vi "FPGA_TANK_PRESS.vi"() -> ()   [LabVIEW 2018]
uses:
  <vilib>/LabVIEW Targets/FPGA/cRIO/shared/nicrio_ModuleControls/nicrio_cRIO-9205_VoltageRange.ctl
  <vilib>/LabVIEW Targets/FPGA/cRIO/shared/nicrio_ModuleControls/nicrio_cRIO-9205_TerminalMode.ctl
  <vilib>/rvi/Emulation/niFpgaGetClockAttributes.vi
  <vilib>/rvi/Emulation/niFpgaSctlEmulationGetInTimedLoop.vi
  <vilib>/rvi/Emulation/niFpgaEmulationReportErrorSimple.vi
  <vilib>/rvi/eio/common/nirviEmuTemplateMethod_errors.vi
  <vilib>/rvi/interface/RandomDataEmulation/niFpgaRandomDataHandleErrors.vi
  <vilib>/rvi/Emulation/niFpgaCriticalErrorInLSC.vi
  <vilib>/eio/EIOMethodNode/EIOMethodNode.xnode
  <vilib>/eio/EIONode/EIONode.xnode
  <vilib>/rvi/DataTransferAndStorage/Container/XNode/niFpgaContainer.xnode
  <vilib>/rvi/interface/RandomDataEmulation/nirviRandomDataFpgaReadWriteTemplate.vi
panel:
  out "Mod1/AI3":fxp<+/-,26,5>
  out "Mod1/AI2":fxp<+/-,26,5>
  out "Mod1/AI1":fxp<+/-,26,5>
  in  "Loop Rate (uS) 2":u32=4000
  out "Mod1/DI0":bool
  in  "Mod1/DO0 2":bool
  out "Mod1/AI0":fxp<+/-,26,5>
  in  "stop":bool
  out "FPGA Error Out 2":errorcluster
  in  "Mod2/DO0":bool
  in  "Mod2/DO3":bool
  in  "Mod2/DO2":bool
  in  "Mod2/DO1":bool
  in  "Mod2/DO4":bool
  in  "Mod2/DO7":bool
  in  "Mod2/DO6":bool
  in  "Mod2/DO5":bool
  in  "Stop":bool
  in  "Loop Rate (uS)":u32
  out "FPGA Error Out":errorcluster
  out "Data FIFO Full":bool
  in  "Update AI Settings":bool
  in  "AI Channel Settings":T3(array[cluster])=[{"Voltage Range"=enum."+/- 10V", "Terminal Mode"=enum."RSE"}, {"Voltage Range"=enum."+/- 10V", "Terminal Mode"=enum."RSE"}, {"Voltage Range"=enum."+/- 10V", "Terminal Mode"=enum."RSE"}, {"Voltage Range"=enum."+/- 10V", "Terminal Mode"=enum."RSE"}]
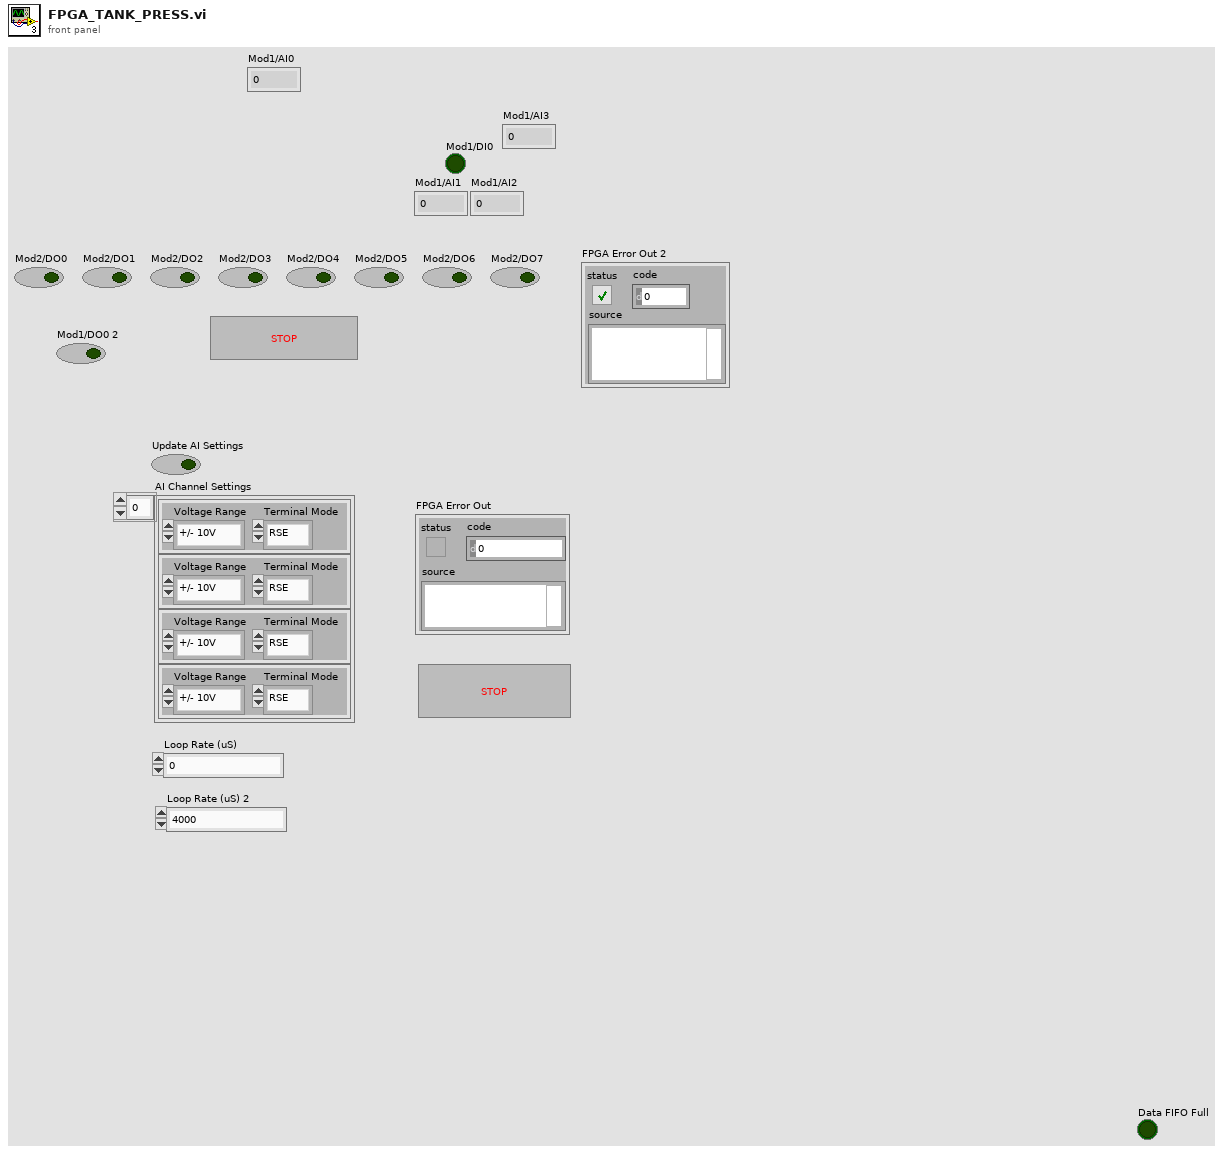
[diagram p1: front panel]
types:
  T1 = typedef "nicrio_cRIO-9205_VoltageRange.ctl" = enum8{"+/- 10V", "+/- 5V", "+/- 1V", "+/- 200mV"}
  T2 = typedef "nicrio_cRIO-9205_TerminalMode.ctl" = enum8{"RSE", "NRSE", "DIFF"}
  T3 = cluster{"Voltage Range":T1, "Terminal Mode":T2}[]
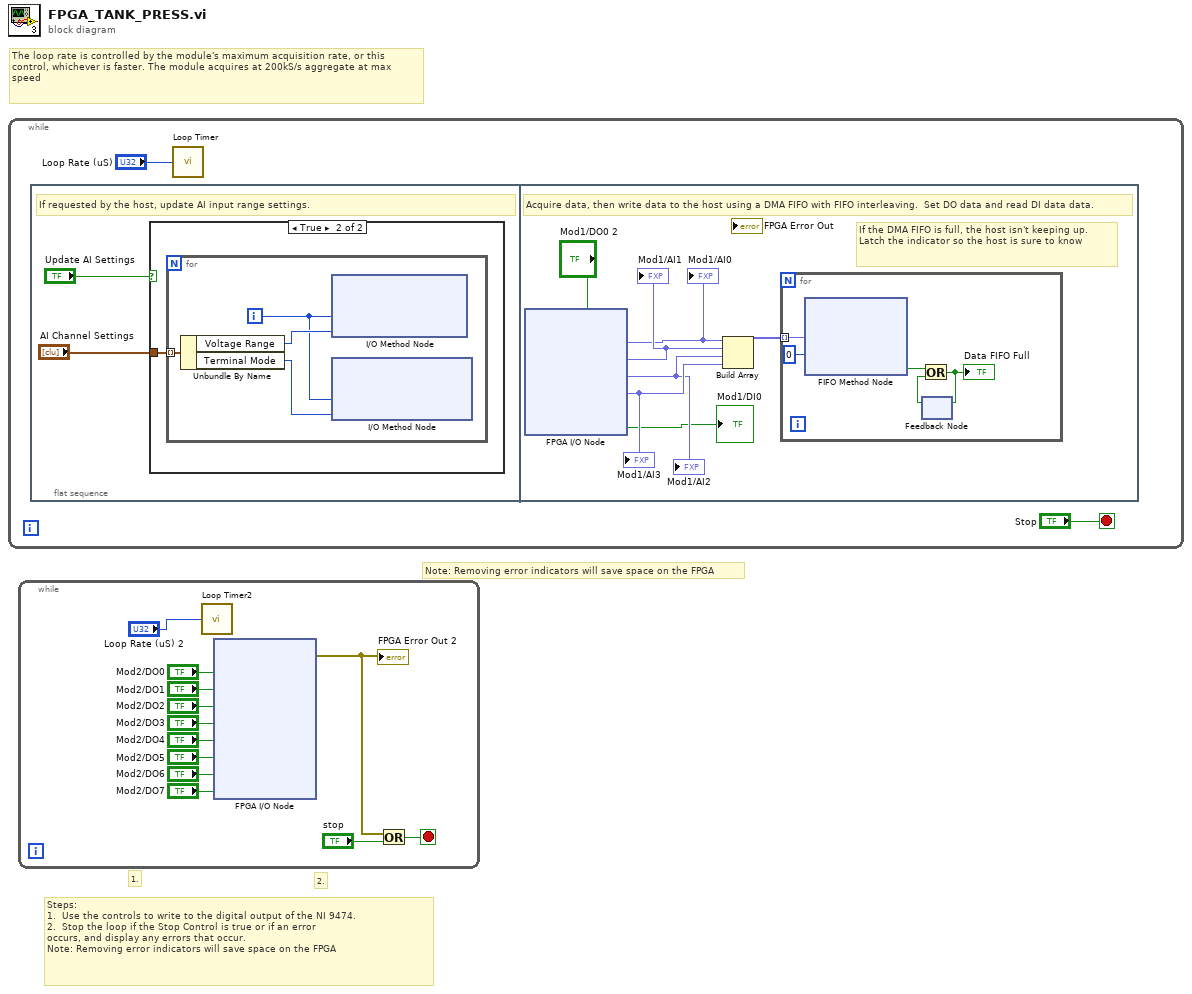
[diagram p0: block diagram]
diagram:
  # "2."
  # "1."
  # "Steps: \n1.  Use the controls to write to the digital output of the NI 9474. \n2.  Stop the loop if the Stop Control is true or if an error\noccurs, and display any errors that occur. \nNote: Removing error indicators will save space on the FPGA"
  # "Note: Removing error indicators will save space on the FPGA"
  # "The loop rate is controlled by the module's maximum acquisition rate, or this control, whichever is faster. The module acquires at 200kS/s aggregate at max speed"
  n1 = while {
    stop <- "Stop" stop-if-true
    n2 = flat-sequence {
      frame #0 {
        # "If requested by the host, update AI input range settings."
        n3 = case shown="True" "Update AI Settings" {
          tunnel: "AI Channel Settings" -> [_ w5]
          frame False {
          }
          frame True {
            n4 = for {
              tunnel: w5 -> [w9] mode=indexing
              i -> [w6]
              n5 = Unbundle By Name(w9) -> ("Voltage Range"=w7:T1, "Terminal Mode"=w8:T2)
              n6 = xnode "I/O Method Node"("AI Channel"=w6, "Voltage Range"=w7) -> ()  [unwired: 1 in, 1 out]
              n7 = xnode "I/O Method Node"("AI Channel"=w6, "Terminal Mode"=w8) -> ()  [unwired: 1 in, 1 out]
            }
          }
        }
      }
      frame #1 {
        # "If the DMA FIFO is full, the host isn't keeping up. \nLatch the indicator so the host is sure to know"
        # "Acquire data, then write data to the host using a DMA FIFO with FIFO interleaving.  Set DO data and read DI data data."
        n8 = xnode "FPGA I/O Node"("Mod1/DO0"="Mod1/DO0 2") -> ("Mod1/AI0"=w13:fxp<+/-,26,5>, "Mod1/AI1"=w14:fxp<+/-,26,5>, "Mod1/AI2"=w15:fxp<+/-,26,5>, "Mod1/AI3"=w16:fxp<+/-,26,5>, "Mod1/DI0"=→"Mod1/DI0":bool)  [unwired: 7 in, 7 out]
        "Mod1/AI0" <- w13
        "Mod1/AI1" <- w14
        "Mod1/AI2" <- w15
        "Mod1/AI3" <- w16
        n9 = Build Array(w13, w14, w15, w16) -> (w12:fxp<+/-,26,5>[])
        n10 = for {
          tunnel: w12 -> [w21] mode=indexing
          n11 = xnode ("FIFO Method Node")("Element"=w21, "Timeout"=0) -> ("Timed Out?"=w17:bool)  [unwired: 1 in, 1 out]
          n12 = feedback #1() -> (w19:bool)  [unwired: 1 out]
          n13 = Or(x=w17, y=w19) -> (x .or. y?=w18:bool)
          "Data FIFO Full" <- w18
          n14 = feedback-in #1(w18) -> ()
        }
      }
    }
    n15 = call "Loop Timer"("Count(uSec)"="Loop Rate (uS)") -> ()  [unwired: 1 out]
  }
  n16 = while {
    stop <- w33 stop-if-true
    n17 = call "Loop Timer2"("Count(uSec)"="Loop Rate (uS) 2") -> ()  [unwired: 1 out]
    n18 = xnode "FPGA I/O Node"("Mod2/DO0"="Mod2/DO0", "Mod2/DO0"="Mod2/DO1", "Mod2/DO2"="Mod2/DO2", "Mod2/DO3"="Mod2/DO3", "Mod2/DO4"="Mod2/DO4", "Mod2/DO5"="Mod2/DO5", "Mod2/DO6"="Mod2/DO6", "Mod2/DO7"="Mod2/DO7") -> ("error out"=w31:errorcluster)  [unwired: 9 in, 8 out]
    "FPGA Error Out 2" <- w31
    n19 = Or(x=w31, y="stop") -> (x .or. y?=w33:bool)
  }
